vi "题1.vi"() -> ()   [LabVIEW 2017]
panel:
  out "倒计时":string
  in  "停止":bool
  out "布尔":bool
  in  "开始倒计时":bool
  in  "定时时间选择":enum16{"20秒", "10秒", "6秒"}(ring)
  # "倒计时器"
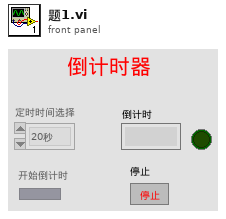
[diagram p1: front panel]
types:
  T1 = enum8{"Enabled", "Disabled", "Disabled and Grayed Out"}
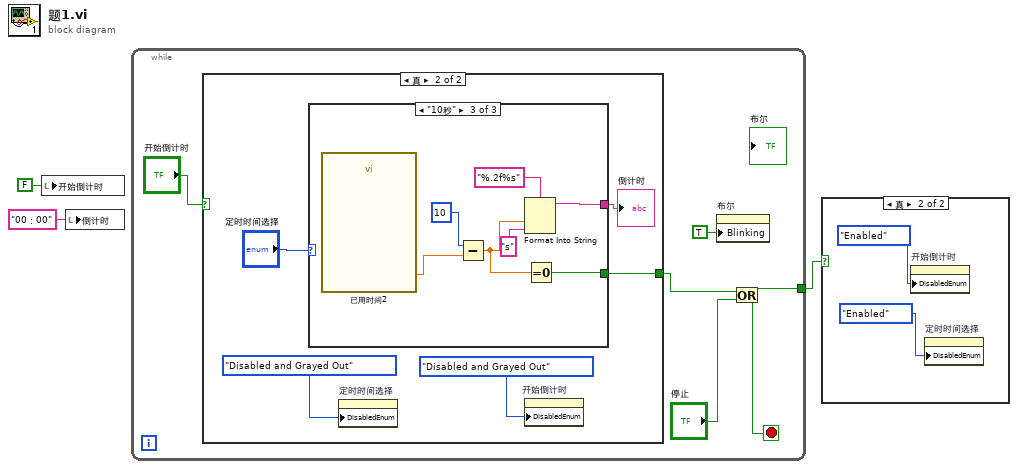
[diagram p0: block diagram]
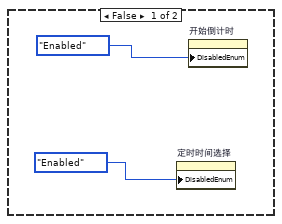
[diagram p3: hidden frame]
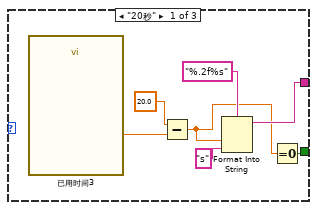
[diagram p4: hidden frame]
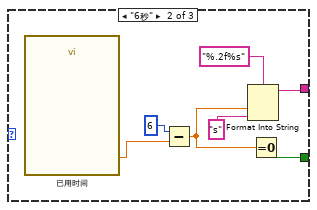
[diagram p5: hidden frame]
diagram:
  n1 = local write "开始倒计时"(FALSE ("开始倒计时")) -> ()
  n2 = local write "倒计时"("00：00" ("倒计时")) -> ()
  n3 = while {
    tunnel: [w5] -> w2
    stop <- w5 stop-if-true
    n4 = case shown="真" "开始倒计时" {
      tunnel: [_ w14] -> w8
      frame False {
        n5 = property on="定时时间选择" class="Enum (严格)"("DisabledEnum"=T1."Enabled" ("禁用")) -> ()  [unwired: 2 in, 2 out]
        n6 = property on="开始倒计时" class="Bool (严格)"("DisabledEnum"=T1."Enabled" ("禁用")) -> ()  [unwired: 2 in, 2 out]
      }
      frame True {
        n7 = case shown="\"10秒\"" "定时时间选择" {
          tunnel: [w17 w24 w31] -> w14
          tunnel: [w18 w23 w30] -> w13
          frame "20秒" {
            n8 = call "已用时间3"() -> ("Elapsed Time (s)"=w22:dbl)  [unwired: 12 in, 7 out]
            n9 = Subtract(x=20.0, y=w22) -> (x-y=w16:dbl)
            n10 = Format Into String(format string="%.2f%s" ("格式字符串"), w16, "s") -> (resulting string=w18:string)  [unwired: 2 in, 1 out]
            n11 = Equal To 0?(x=w16) -> (x = 0?=w17:bool)
          }
          frame "6秒" {
            n12 = call "已用时间"() -> ("Elapsed Time (s)"=w29:dbl)  [unwired: 12 in, 7 out]
            n13 = Subtract(x=6, y=w29) -> (x-y=w25:dbl)
            n14 = Format Into String(format string="%.2f%s" ("格式字符串"), w25, "s") -> (resulting string=w23:string)  [unwired: 2 in, 1 out]
            n15 = Equal To 0?(x=w25) -> (x = 0?=w24:bool)
          }
          frame "10秒" {
            n16 = call "已用时间2"() -> ("Elapsed Time (s)"=w36:dbl)  [unwired: 12 in, 7 out]
            n17 = Subtract(x=10, y=w36) -> (x-y=w32:dbl)
            n18 = Format Into String(format string="%.2f%s" ("格式字符串"), w32, "s") -> (resulting string=w30:string)  [unwired: 2 in, 1 out]
            n19 = Equal To 0?(x=w32) -> (x = 0?=w31:bool)
          }
        }
        "倒计时" <- w13
        n20 = property on="定时时间选择" class="Enum (严格)"("DisabledEnum"=T1."Disabled and Grayed Out" ("禁用")) -> ()  [unwired: 2 in, 2 out]
        n21 = property on="开始倒计时" class="Bool (严格)"("DisabledEnum"=T1."Disabled and Grayed Out" ("禁用")) -> ()  [unwired: 2 in, 2 out]
      }
    }
    n22 = property on="布尔" class="Bool (严格)"("Blinking"=TRUE ("闪烁")) -> ()  [unwired: 2 in, 2 out]
    n23 = Or(x=w8, y="停止") -> (x .or. y?=w5:bool)
  }
  n24 = case shown="真" w2 {
    frame False {
    }
    frame True {
      n25 = property on="开始倒计时" class="Bool (严格)"("DisabledEnum"=T1."Enabled" ("禁用")) -> ()  [unwired: 2 in, 2 out]
      n26 = property on="定时时间选择" class="Enum (严格)"("DisabledEnum"=T1."Enabled" ("禁用")) -> ()  [unwired: 2 in, 2 out]
    }
  }
